vi "signal_simulate.vi"() -> ()   [LabVIEW 2021]
panel:
  in  "Stop":bool
  out "Difference":dynamicdata(graph)
  out "Sum":dynamicdata(graph)
  in  "Frequency 2":dbl(knob) scale=0.0..10.0
  in  "Frequency":dbl(knob) scale=0.0..10.0
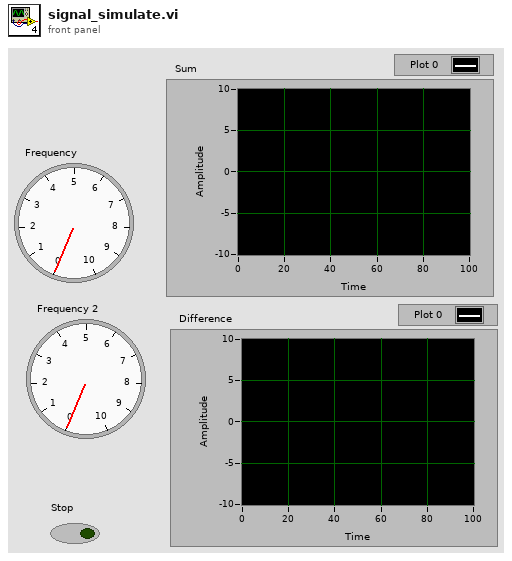
[diagram p1: front panel]
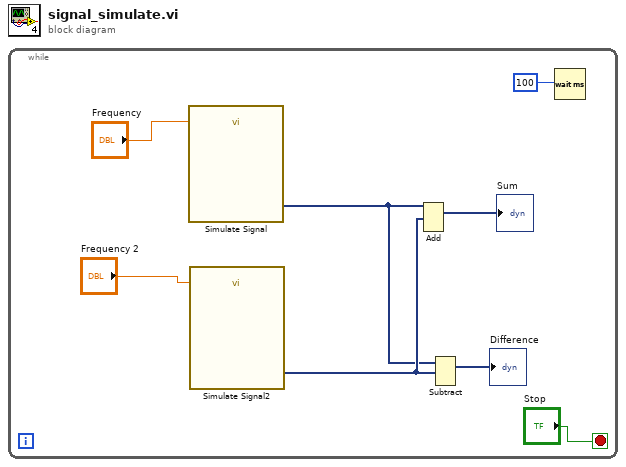
[diagram p0: block diagram]
diagram:
  n1 = while {
    stop <- "Stop" stop-if-true
    n2 = call "Simulate Signal"("Frequency"="Frequency") -> ("Sine with Uniform Noise"=w5:dynamicdata)  [unwired: 13 in, 1 out]
    n3 = call "Simulate Signal2"("Frequency"="Frequency 2") -> ("Square"=w6:dynamicdata)  [unwired: 13 in, 1 out]
    n4 = Add(1:w6, 2:w5) -> (0:→"Sum":dynamicdata)  [unwired: 1 in, 1 out]
    n5 = Subtract(1:w6, 2:w5) -> (0:→"Difference":dynamicdata)  [unwired: 1 in, 1 out]
    n6 = Wait (ms)(milliseconds to wait=100) -> ()  [unwired: 1 out]
  }
